vi "SerializeMessage.vi"(7 "MsgSerializer":refnum<class "MsgSerializer.lvclass">, 9 "error in (no error)":errorcluster, 10 "Value":variant, 11 "TestManagerMsg.CompleteSuite in":refnum<class "TestManagerMsg.CompleteSuite.lvclass">) -> (1 "error out":errorcluster, 3 "Serialized Message":string)   [LabVIEW 2013, in "Caraya.lvlib" / "TestManagerMsg.CompleteSuite.lvclass"]
uses:
  TestManagerMsg.CompleteSuite.lvclass
  MsgSerializer/MsgSerializer.lvclass
  Test Manager Message/TestManagerMsg.lvclass
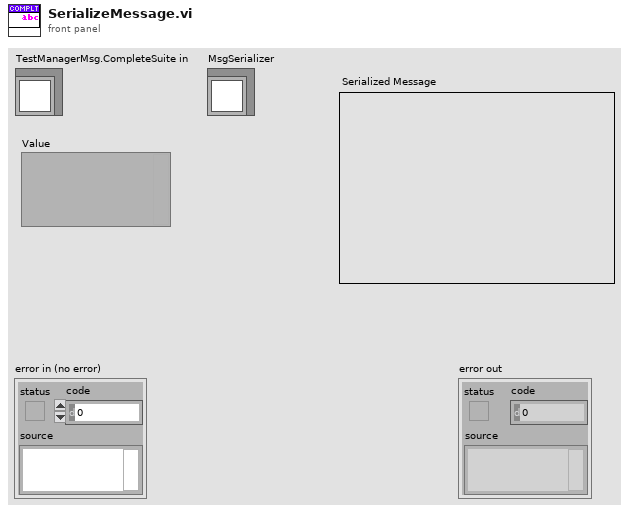
[diagram p1: front panel]
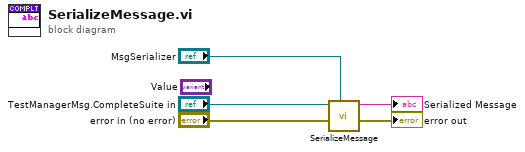
[diagram p0: block diagram]
diagram:
  n1 = call-parent "SerializeMessage.vi"("MsgSerializer"="MsgSerializer", "error in (no error)"="error in (no error)", "TestManagerMsg in"="TestManagerMsg.CompleteSuite in") -> ("error out"=→"error out":errorcluster, "Serialized Message"=→"Serialized Message":string)  [unwired: 7 in]
